vi "WriteData.vi"(8 "Error In":errorcluster, 10 "Data":string, 11 "reference in":refnum<class "DataSourceDecorator.lvclass">) -> (0 "Error Out":errorcluster, 3 "reference out":refnum<class "DataSourceDecorator.lvclass">)   [LabVIEW 2020, in "DataSourceDecorator.lvclass"]
uses:
  DataSourceDecorator.lvclass
  DataSource_interface/DataSource.lvclass
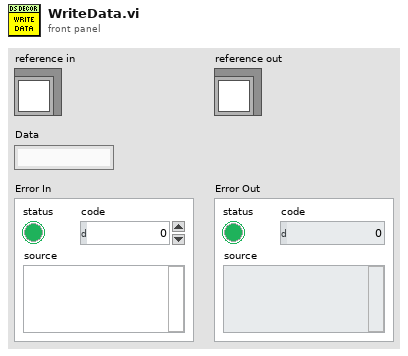
[diagram p1: front panel]
types:
  T1 = typedef "DataSourceDecorator.lvclass/ObjectAttributes.ctl" = cluster{"Wrappee":refnum<class "DataSource.lvclass">}
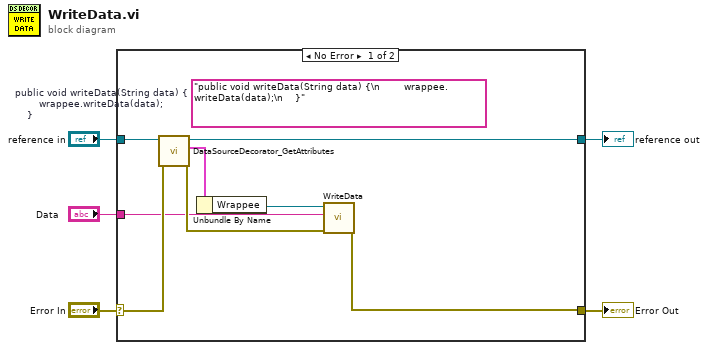
[diagram p0: block diagram]
diagram:
  n1 = case shown="No Error" "Error In" {
    selector: "Error In" -> [w12 w15]
    tunnel: [w7 w15] -> w4
    tunnel: [w11 w14] -> w2
    tunnel: "reference in" -> [w13 w14]
    tunnel: "Data" -> [w6 _]
    frame No Error {
      (unwired) "public void writeData(String data) {\n        wrappee.writeData(data);\n    }"  # public void writeData(String data) {         wrappee.writeData(data);     }
      n2 = call "DataSourceDecorator_GetAttributes.vi"("error in (no error)"=w12, "reference in"=w13) -> ("error out"=w8:errorcluster, "Data"=w10:T1, "reference out"=w11:refnum<class "DataSourceDecorator.lvclass">)  [unwired: 6 in, 1 out]
      n3 = Unbundle By Name(w10) -> ("Wrappee"=w9:refnum<class "DataSource.lvclass">)
      n4 = call-dynamic "WriteData.vi"("Error In"=w8, "Data"=w6, "object in"=w9) -> ("Error Out"=w7:errorcluster)  [unwired: 7 in, 1 out]
    }
    frame Error {
    }
  }
  "Error Out" <- w4
  "reference out" <- w2
